vi "Write comand Start read.vi"(8 "error in (no error)":errorcluster, 9 "Start read":bool, 10 "Output data format":T1(ring), 11 "VISA Refnum in":refnum<visa-resource-name>) -> (0 "error out":errorcluster, 3 "VISA Refnum out":refnum<visa-resource-name>)   [LabVIEW 2017, in "IL Driver Library.lvlib"]
uses:
  IL Driver Library.lvlib
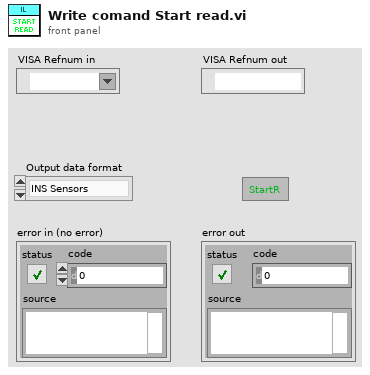
[diagram p1: front panel]
types:
  T1 = enum16{"INS Sensors", "INS OPVT", "INS QPVT", "INS OPVT2A", "INS OPVT2AW", "INS OPVT2Ahr", "INS Minimal", "INS NMEA"}
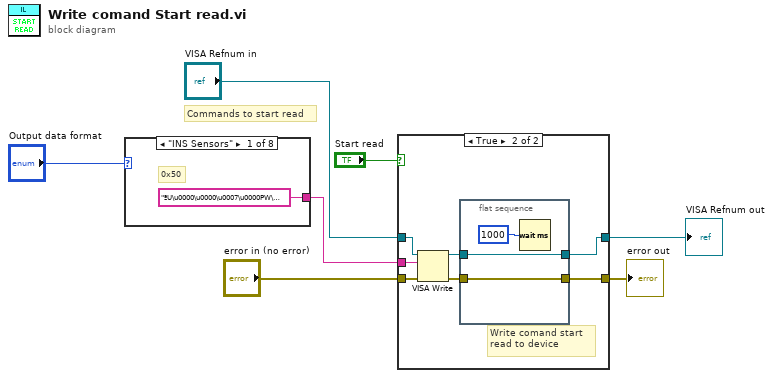
[diagram p0: block diagram]
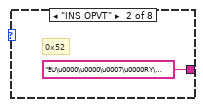
[diagram p2: hidden frame]
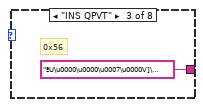
[diagram p3: hidden frame]
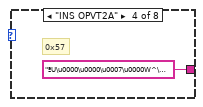
[diagram p4: hidden frame]
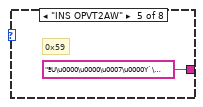
[diagram p5: hidden frame]
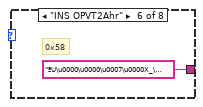
[diagram p6: hidden frame]
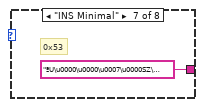
[diagram p7: hidden frame]
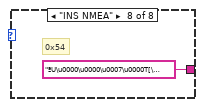
[diagram p8: hidden frame]
diagram:
  # "Commands to start read"
  n1 = case shown="\"INS Sensors\"" "Output data format" {
    tunnel: ["ªU\u0000\u0000\u0007\u0000PW\u0000" ("write buffer") "ªU\u0000\u0000\u0007\u0000RY\u0000" ("write buffer") "ªU\u0000\u0000\u0007\u0000V]\u0000" ("write buffer") "ªU\u0000\u0000\u0007\u0000W^\u0000" ("write buffer") "ªU\u0000\u0000\u0007\u0000Y`\u0000" ("write buffer") "ªU\u0000\u0000\u0007\u0000X_\u0000" ("write buffer") "ªU\u0000\u0000\u0007\u0000SZ\u0000" ("write buffer") "ªU\u0000\u0000\u0007\u0000T[\u0000" ("write buffer")] -> w1
    frame "INS Sensors" {
      # "0x50"
    }
    frame "INS OPVT" {
      # "0x52"
    }
    frame "INS QPVT" {
      # "0x56"
    }
    frame "INS OPVT2A" {
      # "0x57"
    }
    frame "INS OPVT2AW" {
      # "0x59"
    }
    frame "INS OPVT2Ahr" {
      # "0x58"
    }
    frame "INS Minimal" {
      # "0x53"
    }
    frame "INS NMEA" {
      # "0x54"
    }
  }
  n2 = case shown="True" "Start read" {
    tunnel: "VISA Refnum in" -> [w16 w24]
    tunnel: "error in (no error)" -> [w17 w23]
    tunnel: [w16 w20] -> w4
    tunnel: [w17 w19] -> w5
    tunnel: w1 -> [_ w18]
    frame False {
    }
    frame True {
      # "Write comand start \nread to device"
      n3 = VISA Write(VISA resource name=w24, write buffer=w18, error in (no error)=w23) -> (VISA resource name out=w21:refnum<visa-resource-name>, error out=w22:errorcluster)  [unwired: 1 out]
      n4 = flat-sequence {
        tunnel: [w27] -> w19
        tunnel: w22 -> [w27]
        tunnel: w21 -> [w26]
        tunnel: [w26] -> w20
        frame #0 {
          n5 = Wait (ms)(milliseconds to wait=u32 1000) -> ()  [unwired: 1 out]
        }
      }
    }
  }
  "error out" <- w5
  "VISA Refnum out" <- w4
